vi "main.vi"() -> ()   [LabVIEW 2014, in "Janga.lvrbt"]
uses:
  Janga.lvrbt
panel:
  in  "Stop":bool
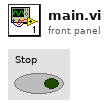
[diagram p1: front panel]
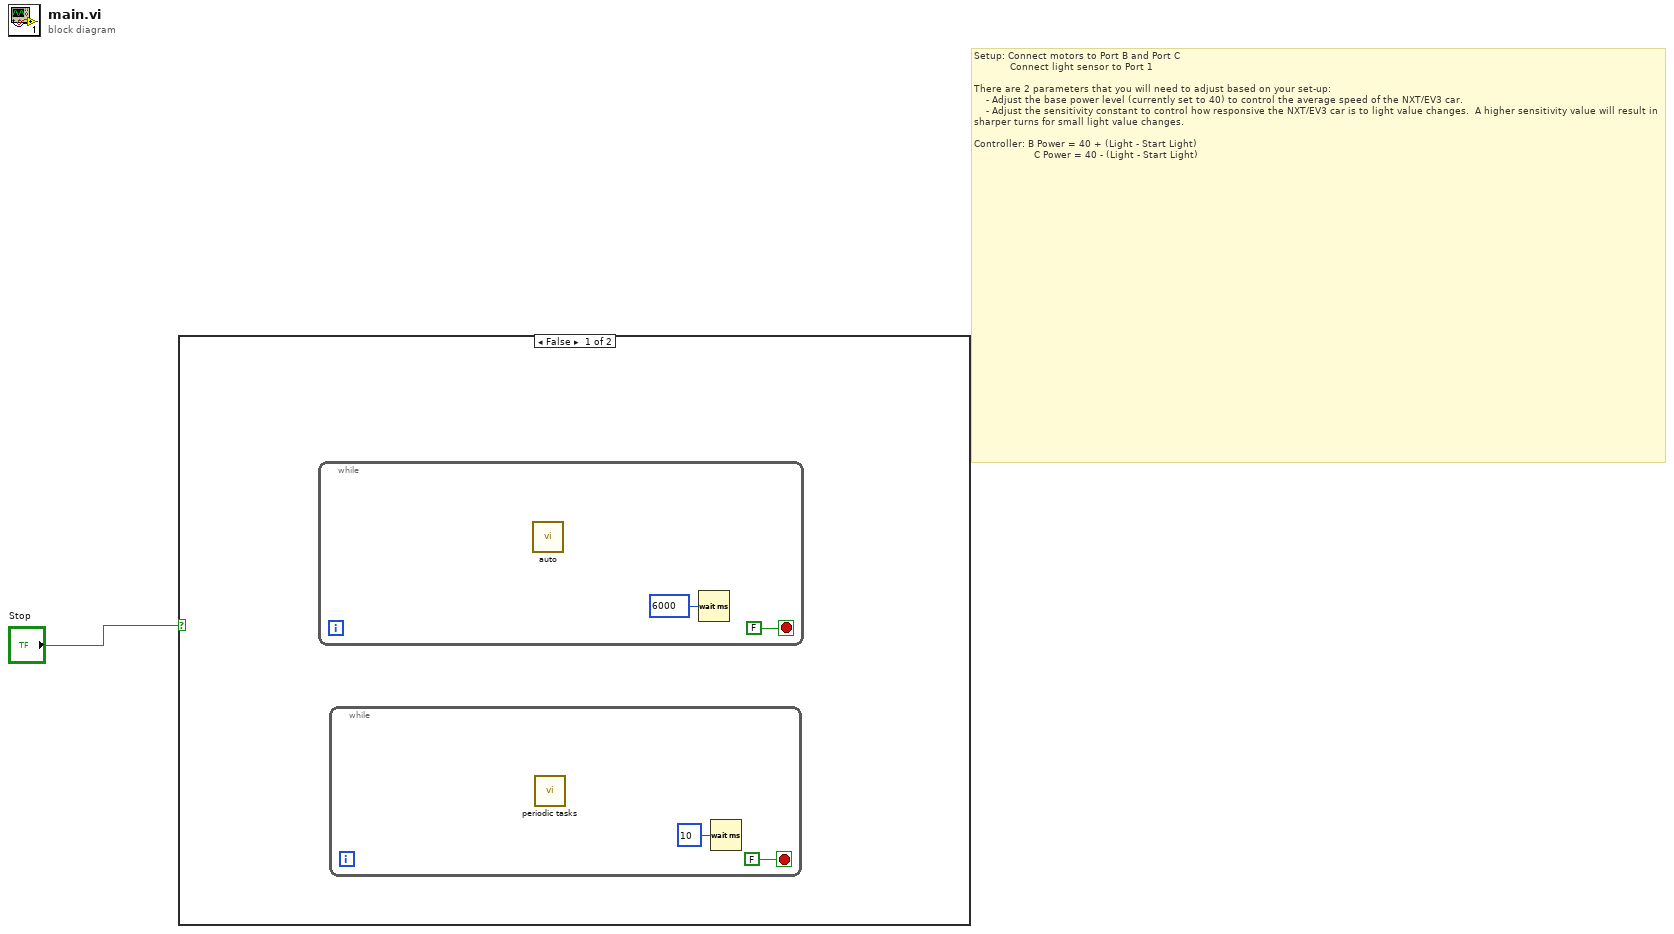
[diagram p0: block diagram]
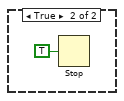
[diagram p2: hidden frame]
diagram:
  # "Setup: Connect motors to Port B and Port C\n            Connect light sensor to Port 1\n\nThere are 2 parameters that you will need to adjust based on your set-up:  \n    - Adjust the base power level (currently set to 40) to control the average speed of the NXT/EV3 car.\n    - Adjust the sensitivity constant to control how responsive the NXT/EV3 car is to light value changes.  A higher sensitivity value will result in sharper turns for small light value changes. \n \nController: B Power = 40 + (Light - Start Light)\n                    C Power = 40 - (Light - Start Light)"
  n1 = case shown="False" "Stop" {
    frame False {
      n2 = while {
        stop <- FALSE stop-if-true
        n3 = call "auto.vi"() -> ()  [unwired: 12 in]
        n4 = Wait (ms)(milliseconds to wait=u32 6000) -> ()  [unwired: 1 out]
      }
      n5 = while {
        stop <- FALSE stop-if-true
        n6 = call "periodic tasks.vi"() -> ()  [unwired: 12 in]
        n7 = Wait (ms)(milliseconds to wait=u32 10) -> ()  [unwired: 1 out]
      }
    }
    frame True {
      n8 = Stop(stop? (T)=TRUE) -> ()
    }
  }
